vi "onTimeout.vi"(8 "error in (no error)":errorcluster, 11 "Last sent message in":refnum<class "BaseMessage.lvclass">) -> (0 "error out":errorcluster, 2 "response":T1, 3 "Last sent message out":refnum<class "BaseMessage.lvclass">)   [LabVIEW 2013, in "BaseMessage.lvclass"]
doc: "Formats a timeout response"
uses:
  BaseMessage.lvclass
  response.ctl
  driver_status.ctl
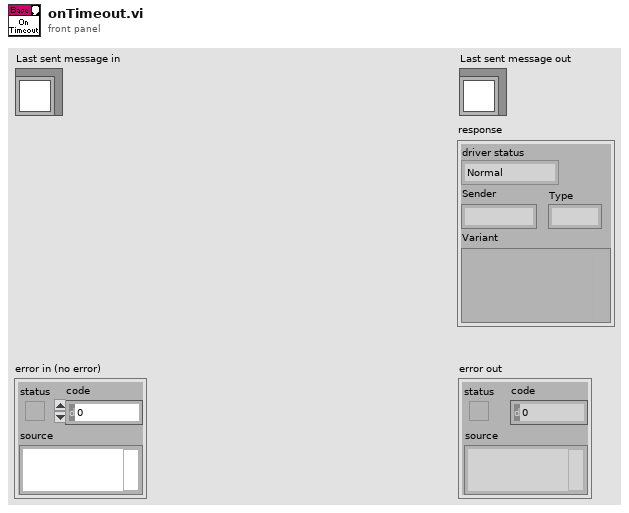
[diagram p1: front panel]
types:
  T1 = typedef "response.ctl" = cluster{"driver status":T2, "Sender":string, "Type":i32, "Variant":variant}
  T2 = typedef "driver_status.ctl" = enum16{"Normal", "Startup", "Connection lost", "Reconnected", "Timeout", "Idle", "Busy"}
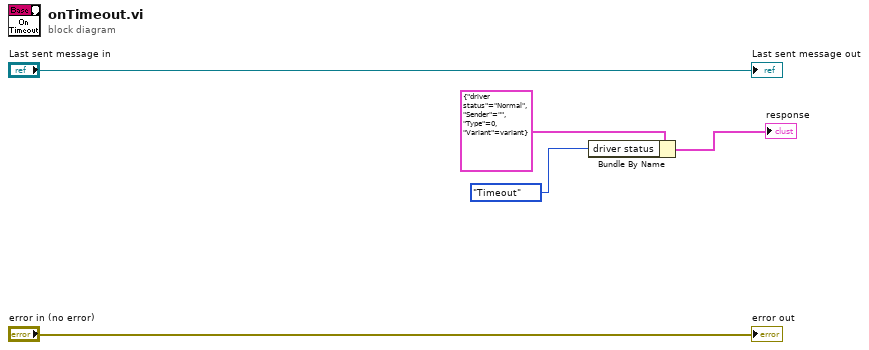
[diagram p0: block diagram]
diagram:
  n1 = Bundle By Name(cluster=T1 {"driver status"=enum."Normal", "Sender"="", "Type"=0, "Variant"=variant} ("response"), "driver status"=driver_status."Timeout") -> (→"response":T1)
  "error out" <- "error in (no error)"
  "Last sent message out" <- "Last sent message in"
